vi "FCGI server.vi"(9 "worker pool size":i32=40, 10 "connection handler pool size":i32=10, 11 "port":u16=4000) -> (0 "error out":errorcluster)   [LabVIEW 2013]
uses:
  worker package.ctl
  application request.ctl
  FCGI begin request role.ctl
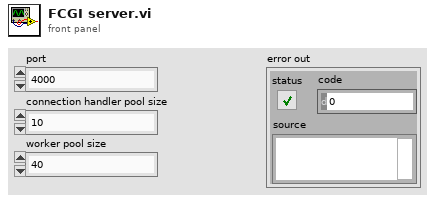
[diagram p1: front panel]
types:
  T1 = typedef "worker package.ctl" = cluster{"TCP Connection":refnum<k5>, "application request":T2}
  T2 = typedef "application request.ctl" = cluster{"request id":u16, "role":T3, "standard input":string, "data":string, "dictionary":variant, "close after response":bool}
  T3 = typedef "FCGI begin request role.ctl" = enum16{"none", "Responder", "Authorizer", "Filter"}
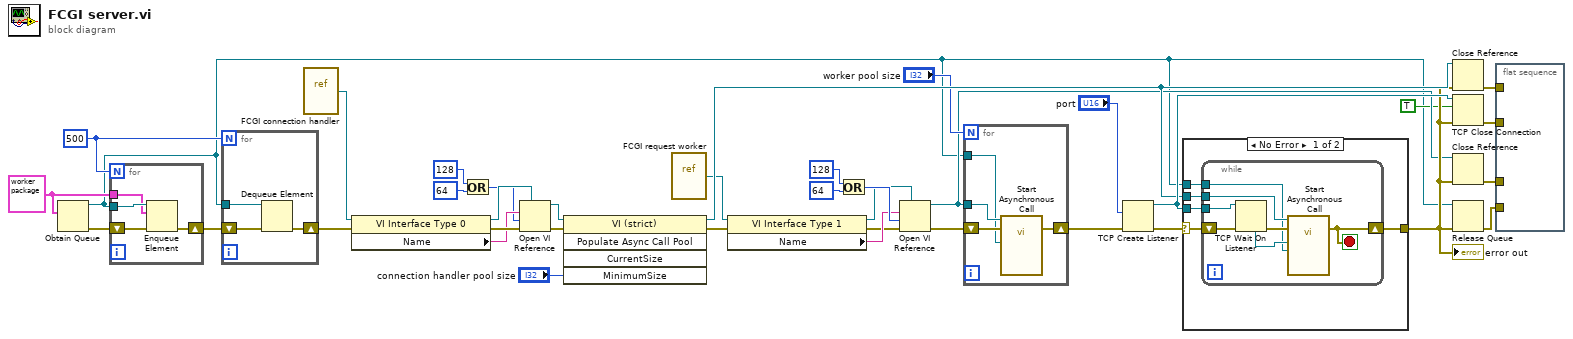
[diagram p0: block diagram]
diagram:
  w2 = 500
  w3 = T1 {"TCP Connection"=refnum, "application request"={"request id"=0, "role"=enum."none", "standard input"="", "data"="", "dictionary"=variant(cluster{"key":string, "value":string}[] []), "close after response"=FALSE}} ("request package")
  n1 = Obtain Queue(element data type=w3) -> (queue out=w1:refnum<queue>, error out=w6:errorcluster)  [unwired: 4 in, 1 out]
  n2 = for {
    N: w2 -> [_]
    shift-right: [w40] -> w5
    shift-left: w6 -> [w41]
    tunnel: w1 -> [w42]
    tunnel: w3 -> [w39]
    n3 = Enqueue Element(queue=w42, element=w39, error in (no error)=w41) -> (error out=w40:errorcluster)  [unwired: 1 in, 2 out]
  }
  n4 = for {
    N: w2 -> [_]
    shift-right: [w44] -> w4
    shift-left: w5 -> [w45]
    tunnel: w1 -> [w43]
    n5 = Dequeue Element(queue=w43, error in (no error)=w45) -> (error out=w44:errorcluster)  [unwired: 1 in, 3 out]
  }
  n6 = vi-ref "FCGI connection handler.vi"() -> (w34:refnum<vi>)
  n7 = property class="VI Interface Type 0"(reference=w34, error in=w4) -> (reference out=w29:refnum<vi>, error out=w33:errorcluster, "Name"=w30:string)
  n8 = Or(x=128 ("options"), y=64 ("options")) -> (x .or. y?=w27:i32)
  n9 = Open VI Reference(type specifier VI Refnum (for type only)=w29, vi path=w30, options=w27, error in (no error)=w33) -> (vi reference=w25:refnum<vi>, error out=w31:errorcluster)  [unwired: 2 in]
  n10 = invoke class="VI (strict)" method="Populate Async Call Pool"(reference=w25, error in=w31, "MinimumSize"="connection handler pool size") -> (reference out=w24:refnum<vi>, error out=w15:errorcluster)  [unwired: 2 in, 3 out]
  n11 = vi-ref "FCGI request worker.vi"() -> (w16:refnum<vi>)
  n12 = property class="VI Interface Type 1"(reference=w16, error in=w15) -> (reference out=w20:refnum<vi>, error out=w18:errorcluster, "Name"=w19:string)
  n13 = Or(x=128 ("options"), y=64 ("options")) -> (x .or. y?=w22:i32)
  n14 = Open VI Reference(type specifier VI Refnum (for type only)=w20, vi path=w19, options=w22, error in (no error)=w18) -> (vi reference=w8:refnum<vi>, error out=w10:errorcluster)  [unwired: 2 in]
  n15 = for {
    N: "worker pool size" -> [_]
    shift-right: [w48] -> w11
    shift-left: w10 -> [w49]
    tunnel: w8 -> [w47]
    tunnel: w1 -> [w46]
    n16 = call-by-ref "Start Asynchronous Call"(reference=w47, error in=w49, "exec queue"=w46) -> (error out=w48:errorcluster)  [unwired: 11 in, 1 out]
  }
  n17 = TCP Create Listener(8:w11, 10:"port") -> (0:w37:errorcluster, 3:w35:refnum<k5>)  [unwired: 3 in, 1 out]
  n18 = case shown="No Error" w37 {
    selector: w37 -> [w54 w62]
    tunnel: [w53 w62] -> w12
    tunnel: w35 -> [w52 _]
    tunnel: w24 -> [w51 _]
    tunnel: w1 -> [w50 _]
    frame No Error {
      n19 = while {
        shift-right: [w58] -> w53
        shift-left: w54 -> [w61]
        tunnel: w52 -> [w60]
        tunnel: w51 -> [w57]
        tunnel: w50 -> [w55]
        stop <- w58 stop-if-true
        n20 = TCP Wait On Listener(8:w61, 11:w60) -> (0:w59:errorcluster, 4:w56:refnum<k5>)  [unwired: 2 in, 3 out]
        n21 = call-by-ref "Start Asynchronous Call"(reference=w57, error in=w59, "exec queue"=w55, "connection"=w56) -> (error out=w58:errorcluster)  [unwired: 10 in, 1 out]
      }
    }
    frame Error {
    }
  }
  "error out" <- w12
  n22 = Close Reference(reference=w24, error in (no error)=w12) -> (error out=w32:errorcluster)
  n23 = TCP Close Connection(connection ID=w35, abort (F)=TRUE, error in (no error)=w12) -> (error out=w36:errorcluster)  [unwired: 1 out]
  n24 = Close Reference(reference=w8, error in (no error)=w12) -> (error out=w14:errorcluster)
  n25 = Release Queue(queue=w1, error in (no error)=w12) -> (error out=w13:errorcluster)  [unwired: 1 in, 2 out]
  n26 = flat-sequence {
    tunnel: w36 -> [_]
    tunnel: w32 -> [_]
    tunnel: w14 -> [_]
    tunnel: w13 -> [_]
    frame #0 {
    }
  }
